vi "Init UDP Config.vi"(8 "error in (no error)":errorcluster, 9 "Graph Buffer Size":i32, 10 "UDP Data":T1={"Decimation"=1, "UDP Buffer Size"=8192, "History Length"=0.5, "Update Rate"=enum."15 Hz", "Channel Paths"=[], "Channel Names"=[]} {"History Length" min=0.5 step=0.5; "UDP Buffer Size" min=8192 max=65536 step=1; "Decimation" min=1 max=1000000 step=1}, 11 "Workspace anager in":T4) -> (0 "error out":errorcluster, 1 "UDP Stream Configuration":T3, 2 "UDPChannelStreamSession out":T5, 3 "WorkspaceManager out":T4)   [LabVIEW 2013, in "Workspace MultiY Graph.lvlib"]
uses:
  Workspace MultiY Graph.lvlib
  <vilib>/NI Veristand/Execution/Workspace/UDPChannelStreamSession.ctl
  NationalInstruments.VeriStand.ClientAPI
  <vilib>/NI Veristand/Execution/Workspace/WorkspaceAPI.ctl
  UDP Stream Configuration.ctl
  UDP Data.ctl
  Update Rate.ctl
  <vilib>/NI Veristand/Execution/Workspace/NI_VS Workspace ExecutionAPI.lvlib
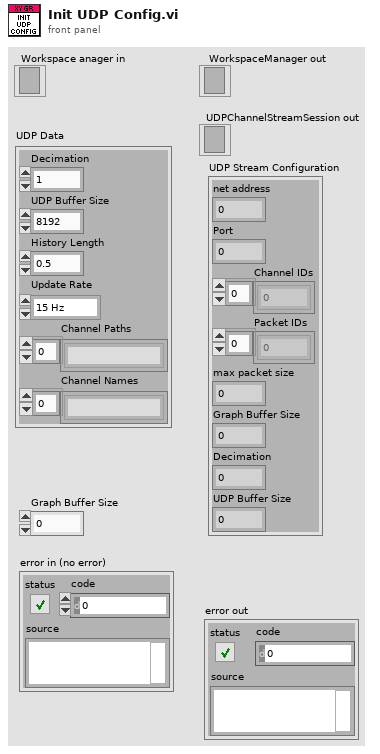
[diagram p1: front panel]
types:
  T1 = typedef "Workspace MultiY Graph.lvlib/UDP Data.ctl" = cluster{"Decimation":i32, "UDP Buffer Size":u32, "History Length":dbl, "Update Rate":T2, "Channel Paths":string[], "Channel Names":string[]}
  T2 = typedef "Workspace MultiY Graph.lvlib/Update Rate.ctl" = enum8{"15 Hz", "10 Hz", "5 Hz", "4 Hz", "3 Hz", "2 Hz", "1 Hz", "0.5 Hz"}
  T3 = typedef "Workspace MultiY Graph.lvlib/UDP Stream Configuration.ctl" = cluster{"net address":u32, "Port":u16, "Channel IDs":i32[], "Packet IDs":i32[], "max packet size":i32, "Graph Buffer Size":i32, "Decimation":i32, "UDP Buffer Size":u32}
  T4 = typedef "NI_VS Workspace ExecutionAPI.lvlib/WorkspaceAPI.ctl" = refnum<k24>
  T5 = typedef "NI_VS Workspace ExecutionAPI.lvlib/UDPChannelStreamSession.ctl" = refnum<k24>
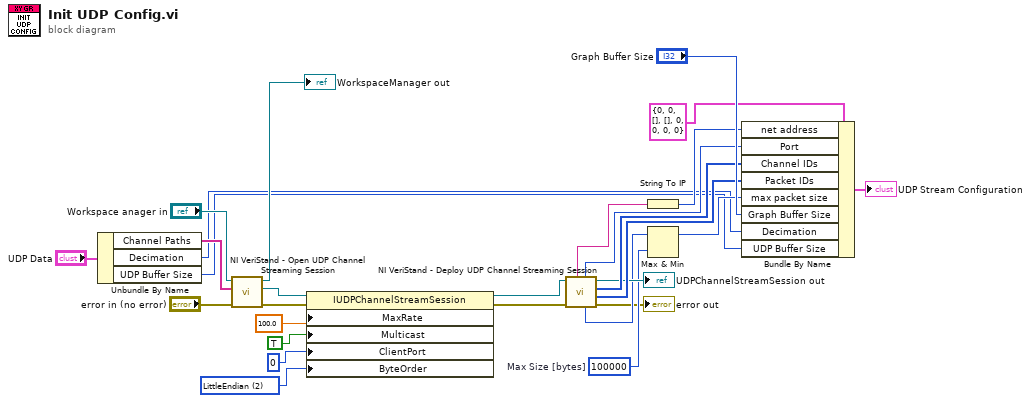
[diagram p0: block diagram]
diagram:
  w3 = 2 items=["BigEndian", "NativeHostOrder", "LittleEndian"] ("ByteOrder")
  w19 = 100000  # Max Size [bytes]
  n1 = Unbundle By Name("UDP Data") -> ("Channel Paths"=w11:string[], "Decimation"=w10:i32, "UDP Buffer Size"=w9:u32)
  n2 = call <vilib>:"NI VeriStand - Open UDP Channel Streaming Session.vi"("error in (no error)"="error in (no error)", "Channels"=w11, "WorkspaceManager in"="Workspace anager in") -> ("error out"=w7:errorcluster, "UDPChannelStreamSession out"=w8:T5, "WorkspaceManager out"=→"WorkspaceManager out":T4)  [unwired: 6 in]
  n3 = property class="IUDPChannelStreamSession"(reference=w8, error in=w7, "MaxRate"=100.0, "Multicast"=TRUE, "ClientPort"=u16 0, "ByteOrder"=w3) -> (reference out=w1:T5, error out=w2:errorcluster)
  n4 = call <vilib>:"NI VeriStand - Deploy UDP Channel Streaming Session.vi"("error in (no error)"=w2, "UDPChannelStreamSession in"=w1) -> ("error out"=→"error out":errorcluster, "Packet IDs"=w26:i32[], "Channel IDs"=w25:i32[], "UDPChannelStreamSession out"=→"UDPChannelStreamSession out":T5, "Max Packet Size"=w20:i32, "Port"=w15:u16, "UDP Multicast Address"=w21:string)  [unwired: 3 in]
  n5 = String To IP(1:w21) -> (0:w16:u32)
  n6 = Max & Min(x=w20, y=w19) -> (max(x,y)=w27:i32)  [unwired: 1 out]
  n7 = Bundle By Name(cluster=T3 {"net address"=0, "Port"=0, "Channel IDs"=[], "Packet IDs"=[], "max packet size"=0, "Graph Buffer Size"=0, "Decimation"=0, "UDP Buffer Size"=0} ("UDP Stream Configuration in"), "net address"=w16, "Port"=w15, "Channel IDs"=w25, "Packet IDs"=w26, "max packet size"=w27, "Graph Buffer Size"="Graph Buffer Size", "Decimation"=w10, "UDP Buffer Size"=w9) -> (→"UDP Stream Configuration":T3)
